vi "getAggregateBounds.vi"(6 "useControlBodyOnly":bool, 8 "error in (no error)":errorcluster, 11 "refs":refnum<vi>[](array[refnum])) -> (0 "error out":errorcluster, 2 "rect":T1, 3 "refs(dup)":refnum<vi>[](array[refnum]))   [LabVIEW 2023, in "TLC_Geometry.lvlib"]
doc: "Calculates the overall bounding rectangle (Top, Left, Bottom, Right) that contains all input controls.\nWhen 'useControlBodyOnly' is enabled, captions and labels are excluded from the calculation."
uses:
  TLC_Geometry.lvlib
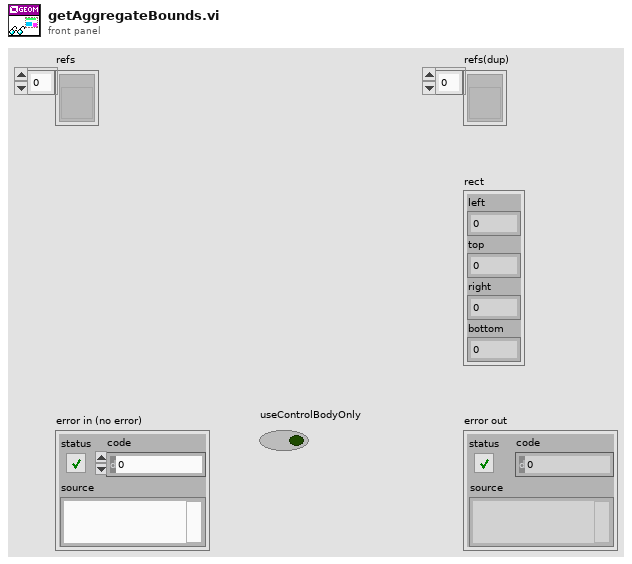
[diagram p1: front panel]
types:
  T1 = cluster{"left":i32, "top":i32, "right":i32, "bottom":i32}
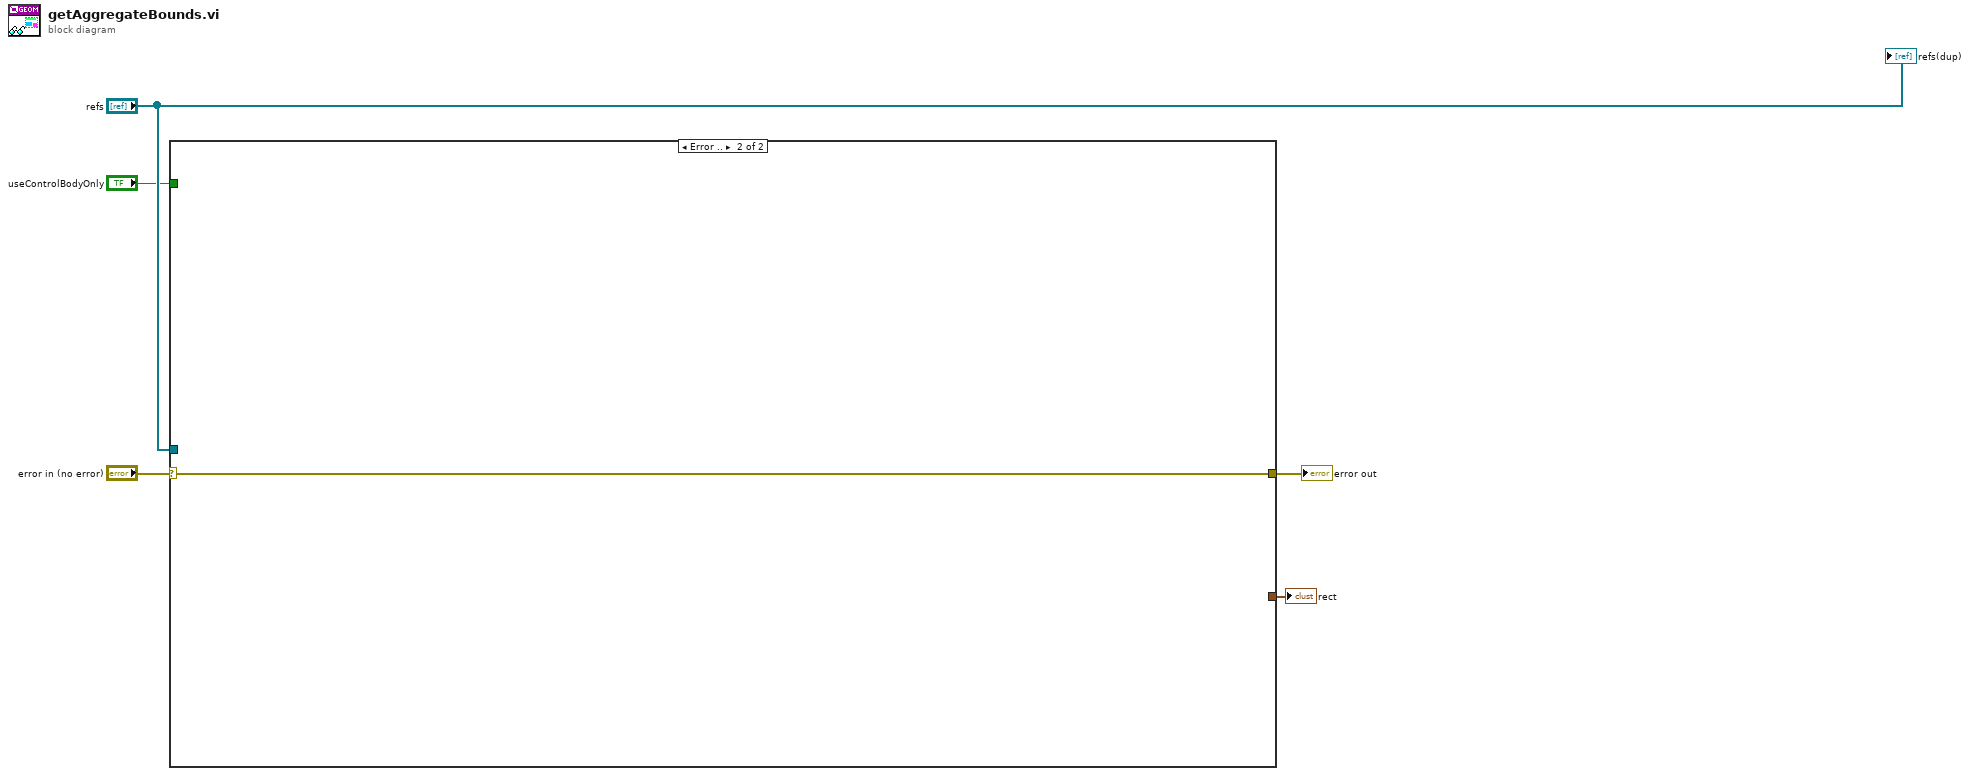
[diagram p0: block diagram]
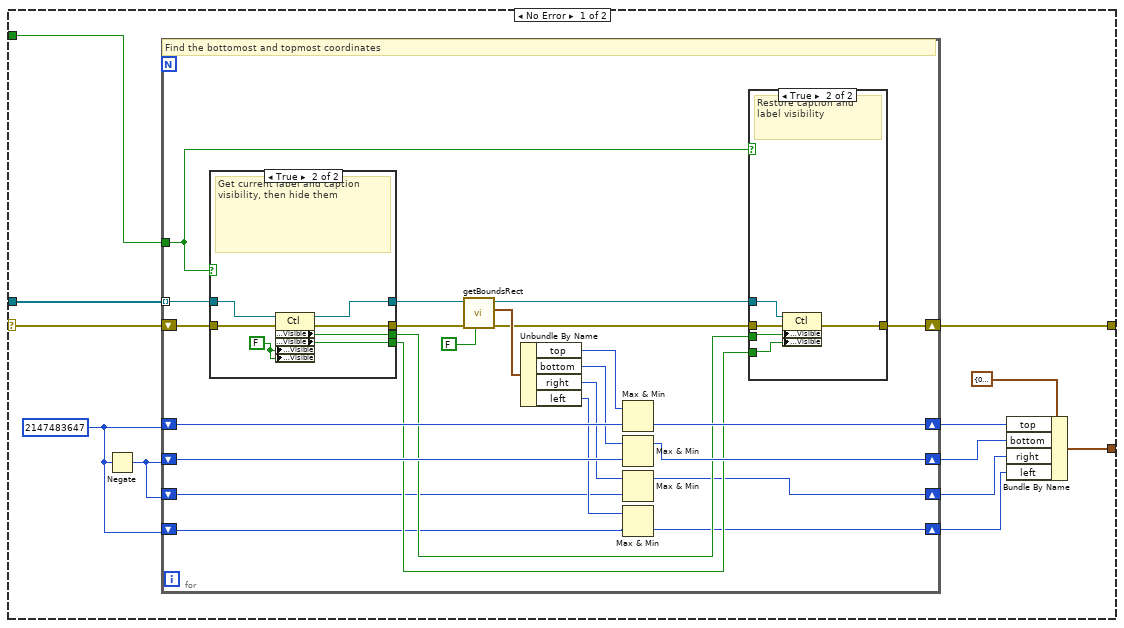
[diagram p2: hidden frame]
diagram:
  n1 = case shown="Error .." "error in (no error)" {
    selector: "error in (no error)" -> [w17 w57]
    tunnel: "refs" -> [w16 _]
    tunnel: "useControlBodyOnly" -> [w15 _]
    tunnel: [w7 _] -> w2
    tunnel: [w6 w57] -> w1
    frame No Error {
      w13 = 2147483647
      n2 = Negate(x=w13) -> (-x=w14:i32)
      n3 = for {
        tunnel: w16 -> [w38] mode=indexing
        shift-right: [w28] -> w6
        shift-left: w17 -> [w37]
        shift-right: [w32] -> w11
        shift-left: w13 -> [w41]
        tunnel: w15 -> [w27]
        shift-right: [w30] -> w10
        shift-left: w14 -> [w34]
        shift-right: [w21] -> w9
        shift-left: w14 -> [w20]
        shift-right: [w19] -> w8
        shift-left: w13 -> [w18]
        # "Find the bottomost and topmost coordinates"
        n4 = case shown="True" w27 {
          tunnel: [w49 w56] -> w39
          tunnel: w38 -> [w49 w55]
          tunnel: w37 -> [w48 w54]
          tunnel: [w48 w53] -> w36
          tunnel: [_ w52] -> w25
          tunnel: [_ w51] -> w24
          frame False {
            # "Do nothing"
          }
          frame True {
            w50 = FALSE ("Caption.Visible")
            # "Get current label and caption visibility, then hide them"
            n5 = property class="Ctl"(reference=w55, error in=w54, "Caption.Visible"=w50, "Label.Visible"=w50) -> (reference out=w56:refnum<vi>, error out=w53:errorcluster, "Caption.Visible"=w52:bool, "Label.Visible"=w51:bool)
          }
        }
        n6 = call "getBoundsRect.vi"("useControlBodyOnly"=FALSE ("ignoreCaption&Labels"), "error in (no error)"=w36, "ref"=w39) -> ("error out"=w29:errorcluster, "rect"=w40:T1, "ref(dup)"=w26:refnum<vi>)  [unwired: 6 in]
        n7 = Unbundle By Name(w40) -> ("top"=w33:i32, "bottom"=w31:i32, "right"=w23:i32, "left"=w22:i32)
        n8 = Max & Min(x=w33, y=w41) -> (min(x,y)=w32:i32)  [unwired: 1 out]
        n9 = Max & Min(x=w31, y=w34) -> (max(x,y)=w30:i32)  [unwired: 1 out]
        n10 = Max & Min(x=w23, y=w20) -> (max(x,y)=w21:i32)  [unwired: 1 out]
        n11 = Max & Min(x=w22, y=w18) -> (min(x,y)=w19:i32)  [unwired: 1 out]
        n12 = case shown="True" w27 {
          tunnel: [w42 w47] -> w28
          tunnel: w29 -> [w42 w46]
          tunnel: w26 -> [_ w45]
          tunnel: w25 -> [_ w44]
          tunnel: w24 -> [_ w43]
          frame False {
            # "Do nothing"
          }
          frame True {
            # "Restore caption and label visibility"
            n13 = property class="Ctl"(reference=w45, error in=w46, "Caption.Visible"=w44, "Label.Visible"=w43) -> (error out=w47:errorcluster)  [unwired: 1 out]
          }
        }
      }
      n14 = Bundle By Name(cluster=T1 {"left"=0, "top"=0, "right"=0, "bottom"=0} ("rect"), "top"=w11, "bottom"=w10, "right"=w9, "left"=w8) -> (w7:T1)
    }
    frame Error {
    }
  }
  "error out" <- w1
  "rect" <- w2
  "refs(dup)" <- "refs"
